vi "Set Initialization Data - subWorker 01.vi"(8 "error in":errorcluster, 11 "Head Worker in":refnum<class "Head Worker.lvclass">) -> (0 "error out":errorcluster, 3 "Head Worker out":refnum<class "Head Worker.lvclass">)   [LabVIEW 2017, in "Head Worker.lvclass"]
doc: "In this VI you can set the initialization data of a statically-linked subWorker."
uses:
  Head Worker.lvclass
  subWorker Level 1/Initialization Data.ctl
  subWorker Level 1/Response Cases.ctl
  Head Worker.lvclass/Head Worker.ctl
  subWorker Level 1/subWorker Level 1.lvclass
  C:/Program Files (x86)/National Instruments/LabVIEW 2017/vi.lib/addons/_Workers/Library/Classes/Worker/Worker.lvclass
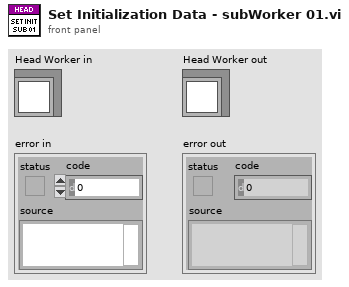
[diagram p1: front panel]
types:
  T1 = typedef "subWorker Level 1.lvclass/Initialization Data.ctl" = cluster{"Response Cases":T2}
  T2 = typedef "subWorker Level 1.lvclass/Response Cases.ctl" = cluster{"Placeholder - Can be deleted":string}
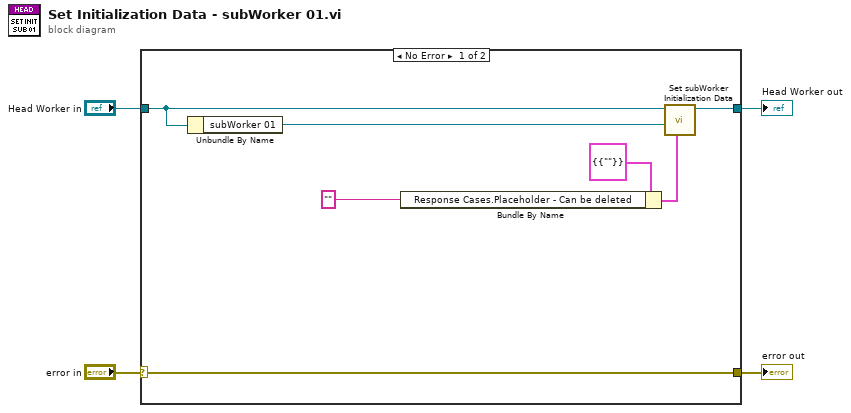
[diagram p0: block diagram]
diagram:
  n1 = case shown="No Error" "error in" {
    selector: "error in" -> [w11 w13]
    tunnel: [w11 w13] -> w3
    tunnel: [w9 w12] -> w2
    tunnel: "Head Worker in" -> [w8 w12]
    frame No Error {
      n2 = Unbundle By Name(w8) -> ("subWorker 01"=w10:refnum<class "subWorker Level 1.lvclass">)
      n3 = Bundle By Name(cluster=T1 {"Response Cases"={"Placeholder - Can be deleted"=""}} ("Initialization Data"), "Response Cases.Placeholder - Can be deleted"="" ("Placeholder")) -> (w6:T1)
      n4 = call-dynamic "Set subWorker Initialization Data.vi"("Initialization Data"=w6, "subWorker"=w10, "Worker"=w8) -> ("Worker out"=w9:refnum<class "Head Worker.lvclass">)  [unwired: 8 in]
    }
    frame Error {
    }
  }
  "error out" <- w3
  "Head Worker out" <- w2
